vi "Test Find Dynamic Dispatch VI in Inheriting lvclass.vi"(8 "error in (no error)":errorcluster, 11 "Test Case In":refnum<class "Interface Identifier Test.lvclass">) -> (0 "error out":errorcluster, 3 "Test Case Out":refnum<class "Interface Identifier Test.lvclass">)   [LabVIEW 2020, in "Interface Identifier Test.lvclass"]
uses:
  Interface Identifier Test.lvclass
  Interface Identifier Test.lvclass/Interface Identifier Test.ctl
  4993e8ee-a06a-463a-9684-69129f64d5ce.vi
  source/Scripting/Interface Identifier/Interface Identifier.lvclass
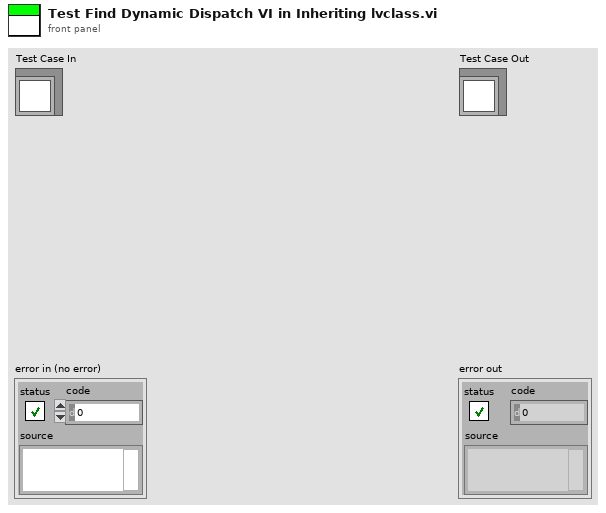
[diagram p1: front panel]
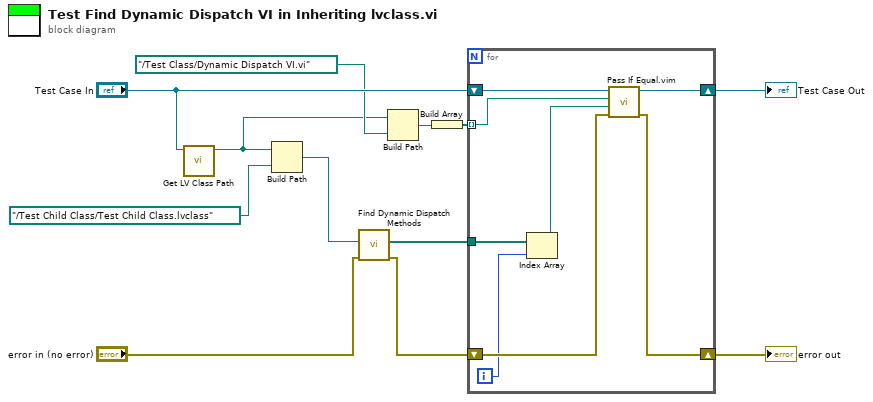
[diagram p0: block diagram]
diagram:
  n1 = call <vilib>:"Get LV Class Path.vi"("object"="Test Case In") -> ("class path"=w1:path)  [unwired: 9 in, 1 out]
  n2 = Build Path(base path=w1, name or relative path=path "../Test Child Class/Test Child Class.lvclass") -> (appended path=w6:path)
  n3 = call "Find Dynamic Dispatch Methods.vi"("error in (no error)"="error in (no error)", "Class Path"=w6) -> ("error out"=w2:errorcluster, "Dynamic Dispatch VIs"=w8:path[])  [unwired: 8 in]
  n4 = Build Path(base path=w1, name or relative path=path "../Test Class/Dynamic Dispatch VI.vi") -> (appended path=w5:path)
  n5 = Build Array(w5) -> (w4:path[])
  n6 = for {
    shift-right: [w18] -> w11
    shift-left: w2 -> [w19]
    shift-right: [w20] -> w12
    shift-left: "Test Case In" -> [w17]
    tunnel: w8 -> [w16]
    tunnel: w4 -> [w15] mode=indexing
    i -> [w13]
    n7 = Index Array(array=w16, index=w13) -> (element=w14:path)
    n8 = call "Pass If Equal.vim"("error in (no error)"=w19, "Actual"=w14, "Expected"=w15, "LUnit Test Case In"=w17) -> ("error out"=w18:errorcluster, "LUnit Test Case Out"=w20:refnum<class "Interface Identifier Test.lvclass">)  [unwired: 6 in]
  }
  "error out" <- w11
  "Test Case Out" <- w12
